vi "SLT Close Process Handle.vi"(0 "handle":i64, 11 "error in (no error)":errorcluster) -> (15 "error out":errorcluster)   [LabVIEW 2013, in "ProcessInfo.lvlib"]
doc: "Closes an open object handle."
uses:
  ProcessInfo.lvlib
  kernel32.dll
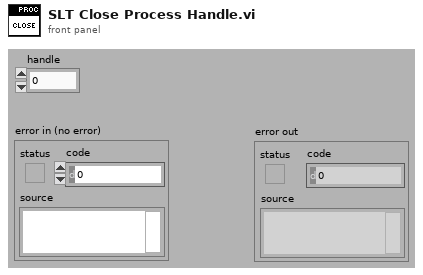
[diagram p1: front panel]
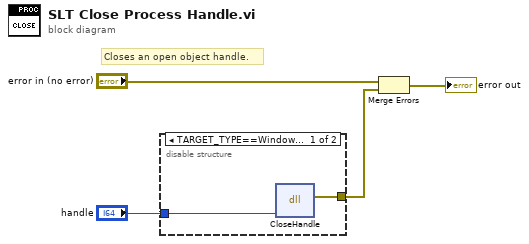
[diagram p0: block diagram]
diagram:
  # "Closes an open object handle."
  n1 = disable-structure shown="TARGET_TYPE==Windows" {
    disable-tunnel: "handle" -> [w6 _]
    disable-tunnel: [w5 _] -> w1
    frame condition #0 (active) {
      n2 = dll-call lib="kernel32.dll" fn="CloseHandle"("handle"=w6) -> (error out=w5:errorcluster)  [unwired: 4 in, 2 out]
    }
    frame condition #1 {
    }
  }
  n3 = Merge Errors("error in (no error)", w1) -> (→"error out":errorcluster)
